vi "Test Get Visible State.vi"(8 "error in (no error)":errorcluster) -> (0 "error out":errorcluster)   [LabVIEW 2013, in "TEST JKI State Machine API.lvlib"]
uses:
  TEST JKI State Machine API.lvlib
  <vilib>/addons/_JKI Toolkits/Caraya/classes/Test/Test.lvclass
  source/JKI SM/JKI SM.lvclass
  <vilib>/addons/_JKI Toolkits/Caraya/classes/Assert/Assert.lvclass
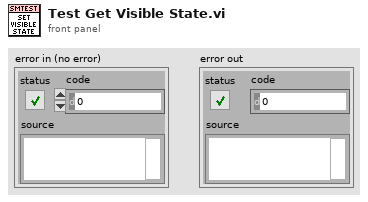
[diagram p1: front panel]
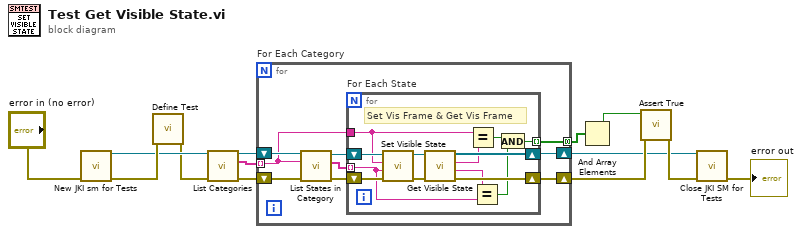
[diagram p0: block diagram]
diagram:
  n1 = call "New JKI sm for Tests.vi"("error in (no error)"="error in (no error)") -> ("error out"=w13:errorcluster, "JKI SM out"=w9:refnum<class "JKI SM.lvclass">)  [unwired: 9 in]
  n2 = call <vilib>:"Define Test.vi"("error in (no error)"=w13) -> ("error out"=w5:errorcluster)  [unwired: 10 in]
  n3 = call "List Categories.vi"("error in (no error)"=w5, "JKI SM in"=w9) -> ("error out"=w6:errorcluster, "All State Categories"=w7:string[], "JKI SM out"=w8:refnum<class "JKI SM.lvclass">)  [unwired: 6 in, 1 out]
  n4 = for "For Each Category" {
    tunnel: w7 -> [w15] mode=indexing
    shift-right: [w19] -> w4
    shift-left: w6 -> [w21]
    shift-right: [w17] -> w3
    shift-left: w8 -> [w22]
    tunnel: [w14] -> w2 mode=concatenating
    n5 = call "List States in Category.vi"("error in (no error)"=w21, "Category"=w15, "JKI SM in"=w22) -> ("error out"=w20:errorcluster, "States"=w16:string[], "JKI SM out"=w18:refnum<class "JKI SM.lvclass">)  [unwired: 4 in, 2 out]
    n6 = for "For Each State" {
      shift-right: [w32] -> w19
      shift-left: w20 -> [w35]
      shift-right: [w30] -> w17
      shift-left: w18 -> [w34]
      tunnel: w16 -> [w27] mode=indexing
      tunnel: w15 -> [w28]
      tunnel: [w23] -> w14 mode=indexing
      # "Set Vis Frame & Get Vis Frame"
      n7 = call "Set Visible State.vi"("error in (no error)"=w35, "State Name"=w27, "Category (Optional)"=w28, "JKI SM in"=w34) -> ("error out"=w33:errorcluster, "JKI SM out"=w31:refnum<class "JKI SM.lvclass">)  [unwired: 6 in]
      n8 = call "Get Visible State.vi"("error in (no error)"=w33, "JKI SM in"=w31) -> ("error out"=w32:errorcluster, "State Name"=w26:string, "Category"=w29:string, "JKI SM out"=w30:refnum<class "JKI SM.lvclass">)  [unwired: 5 in, 1 out]
      n9 = Equal?(x=w28, y=w29) -> (x = y?=w25:bool)
      n10 = Equal?(x=w26, y=w27) -> (x = y?=w24:bool)
      n11 = And(x=w25, y=w24) -> (x .and. y?=w23:bool)
    }
  }
  n12 = And Array Elements(Boolean array=w2) -> (logical AND=w1:bool)
  n13 = call <vilib>:"Assert True.vi"("error in (no error)"=w4, "True?"=w1) -> ("error out"=w11:errorcluster)  [unwired: 9 in]
  n14 = call "Close JKI SM for Tests.vi"("error in (no error)"=w11, "JKI SM in"=w3) -> ("error out"=→"error out":errorcluster)  [unwired: 9 in]
